vi "p15_Temp.vi"() -> ()   [LabVIEW 2022 SP3]
panel:
  in  "Time":dbl(knob) scale=0.0..1000.0
  out "?":dbl(slide) scale=0.0..100.0
  in  "stop":bool
  out "Boolean":bool
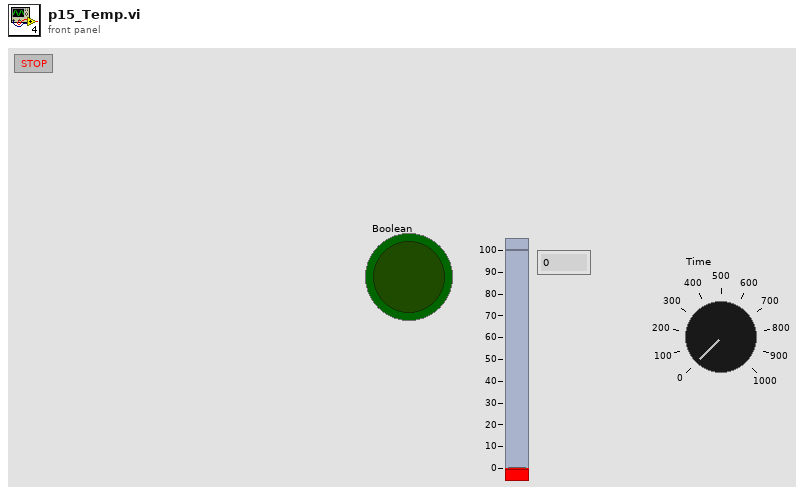
[diagram p1: front panel]
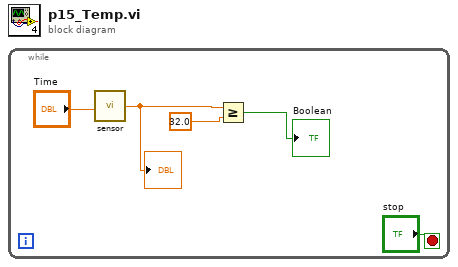
[diagram p0: block diagram]
diagram:
  n1 = while {
    stop <- "stop" stop-if-true
    n2 = call "sensor.vi"("Numeric 2"="Time") -> ("Numeric"=w2:dbl)
    "?" <- w2
    n3 = Greater Or Equal?(x=w2, y=32.0 ("x")) -> (x >= y?=→"Boolean":bool)
  }
